vi "Type Define Ctls.vi"() -> ()   [LabVIEW 2010]
uses:
  Ctrls/PlotGraph.ctl
  Ctrls/Precess Meter.ctl
  Ctrls/ServerData.ctl
  Ctrls/DeviceInfomation.ctl
  Ctrls/DeviceModel.ctl
  Ctrls/ChannelData.ctl
  Ctrls/ChannelType.ctl
  Ctrls/ChannelAccessType.ctl
panel:
  in  "ServerData":T1
  in  "ProcessMeter":T7 {"设定值" format="%07.2f"; "当前值" format="%07.2f"}
  out "Waveform Graph":T8
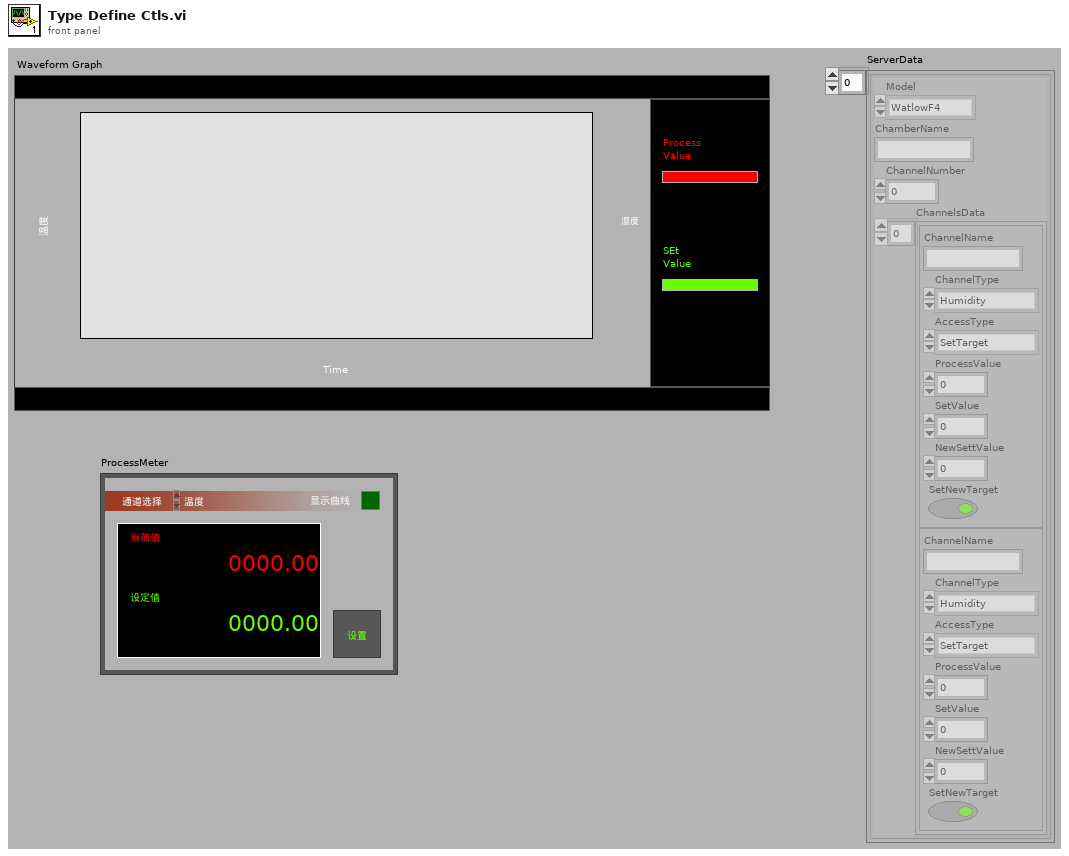
[diagram p1: front panel]
types:
  T1 = typedef "ServerData.ctl" = T2[]
  T2 = typedef "DeviceInfomation.ctl" = cluster{"Model":T3, "ChamberName":string, "ChannelNumber":i32, "ChannelsData":T4[]}
  T3 = typedef "DeviceModel.ctl" = enum16{"WatlowF4", "CenterOne", "DCP551", "DPR250"}
  T4 = typedef "ChannelData.ctl" = cluster{"ChannelName":string, "ChannelType":T5, "AccessType":T6, "ProcessValue":dbl, "SetValue":dbl, "NewSettValue":dbl, "SetNewTarget":bool}
  T5 = typedef "ChannelType.ctl" = enum16{"Temperature", "Humidity"}
  T6 = typedef "ChannelAccessType.ctl" = enum16{"ReadOnly", "SetTarget"}
  T7 = typedef "Precess Meter.ctl" = cluster{"当前值":dbl, "设定值":dbl, "通道选择":enum16{"温度", "湿度"}, "设置设定值":bool, "显示曲线":bool}
  T8 = typedef "PlotGraph.ctl" = dbl[]
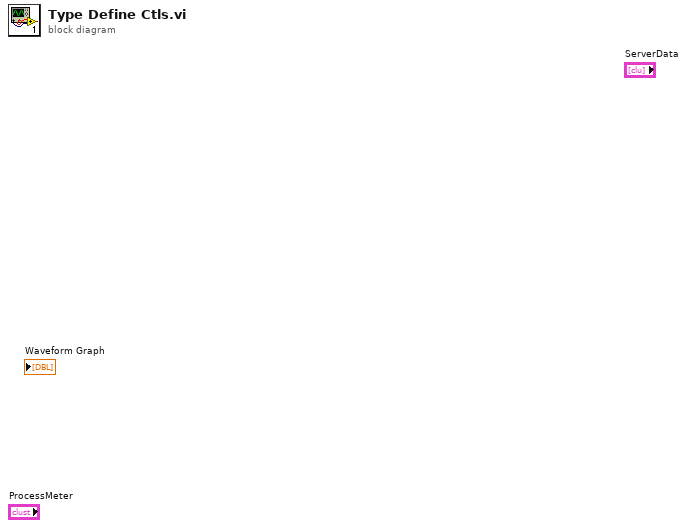
[diagram p0: block diagram]
diagram:
